vi "add_random.vi"() -> ()   [LabVIEW 2021]
uses:
  <vilib>/numeric/Random Number (Range) U64.vi
  <vilib>/numeric/sub_Random U32.vi
panel:
  out "Sum of two dices roll":i32
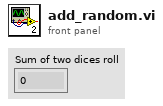
[diagram p1: front panel]
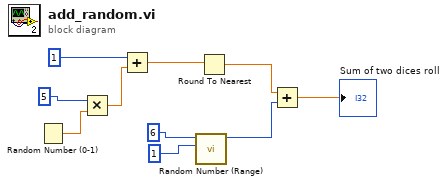
[diagram p0: block diagram]
diagram:
  n1 = Random Number (0-1)() -> (number: 0 to 1=w6:dbl)
  n2 = Multiply(x=5, y=w6) -> (x*y=w10:dbl)
  n3 = Add(x=1, y=w10) -> (x+y=w9:dbl)
  n4 = call-poly <vilib>:"Random Number (Range).vi"("lower bound (0)"=1, "upper bound (100)"=6) -> ("number"=w2:u64)  [unwired: 9 in]
  n5 = Round To Nearest(number=w9) -> (nearest integer value=w3:dbl)
  n6 = Add(x=w3, y=w2) -> (x+y=→"Sum of two dices roll":dbl)
